vi "FindMinimumChiSquaredLMethod.vi"(0 "Extinction ExtinctionUncertainity Size parameter and Number ofS sizes 2":T2={"PAS amplitude"=[7.938e-10, 1.5399999999999999e-09, 2.52e-09, 3.6819999999999995e-09, 4.97e-09, 6.355999999999999e-09], "PAS amp Uncertainty"=[1.21e-11, 5.86e-12, 1.26e-11, 5.3e-11, 1.13e-10, 2.06e-10], "Size parameters"=[1.4957116398663945, 1.869639549832993, 2.243567459799592, 2.61749536976619, 2.991423279732789, 3.3653511896993877], "Number ofSizes"=6.0, "GeometricCrossSection"=[3.1415926535897934e-10, 4.908738521234053e-10, 7.068583470577035e-10, 9.621127501618742e-10, 1.2566370614359174e-09, 1.590431280879833e-09], "Wave Length"=420.07999, "SMPS Sizes"=[181.1, 187.7, 194.6, 200.0, 201.7, 209.1, 216.7, 224.7, 232.9, 241.4, 250.0, 250.3, 259.5, 269.0, 278.8, 289.0, 299.6, 300.0, 310.6, 322.0, 333.8, 346.0, 350.0, 358.7, 371.8, 385.4, 399.5, 400.0, 414.2, 429.4, 445.1, 450.0, 461.4, 478.3, 495.8, 514.0, 532.8, 552.3, 572.5, 593.5, 615.3, 637.8, 661.2, 685.4, 710.5, 736.5, 763.5, 791.5], "Concentration"=[[0.0, 0.0, 0.0, 1.0, 0.0, 0.0, 0.0, 0.0, 0.0, 0.0, 0.0, 0.0, 0.0, 0.0, 0.0, 0.0, 0.0, 0.0, 0.0, 0.0, 0.0, 0.0, 0.0, 0.0, 0.0, 0.0, 0.0, 0.0, 0.0, 0.0, 0.0, 0.0, 0.0, 0.0, 0.0, 0.0, 0.0, 0.0, 0.0, 0.0, 0.0, 0.0, 0.0, 0.0, 0.0, 0.0, 0.0, 0.0], [0.0, 0.0, 0.0, 0.0, 0.0, 0.0, 0.0, 0.0, 0.0, 0.0, 1.0, 0.0, 0.0, 0.0, 0.0, 0.0, 0.0, 0.0, 0.0, 0.0, 0.0, 0.0, 0.0, 0.0, 0.0, 0.0, 0.0, 0.0, 0.0, 0.0, 0.0, 0.0, 0.0, 0.0, 0.0, 0.0, 0.0, 0.0, 0.0, 0.0, 0.0, 0.0, 0.0, 0.0, 0.0, 0.0, 0.0, 0.0], [0.0, 0.0, 0.0, 0.0, 0.0, 0.0, 0.0, 0.0, 0.0, 0.0, 0.0, 0.0, 0.0, 0.0, 0.0, 0.0, 0.0, 1.0, 0.0, 0.0, 0.0, 0.0, 0.0, 0.0, 0.0, 0.0, 0.0, 0.0, 0.0, 0.0, 0.0, 0.0, 0.0, 0.0, 0.0, 0.0, 0.0, 0.0, 0.0, 0.0, 0.0, 0.0, 0.0, 0.0, 0.0, 0.0, 0.0, 0.0], [0.0, 0.0, 0.0, 0.0, 0.0, 0.0, 0.0, 0.0, 0.0, 0.0, 0.0, 0.0, 0.0, 0.0, 0.0, 0.0, 0.0, 0.0, 0.0, 0.0, 0.0, 0.0, 1.0, 0.0, 0.0, 0.0, 0.0, 0.0, 0.0, 0.0, 0.0, 0.0, 0.0, 0.0, 0.0, 0.0, 0.0, 0.0, 0.0, 0.0, 0.0, 0.0, 0.0, 0.0, 0.0, 0.0, 0.0, 0.0], [0.0, 0.0, 0.0, 0.0, 0.0, 0.0, 0.0, 0.0, 0.0, 0.0, 0.0, 0.0, 0.0, 0.0, 0.0, 0.0, 0.0, 0.0, 0.0, 0.0, 0.0, 0.0, 0.0, 0.0, 0.0, 0.0, 0.0, 1.0, 0.0, 0.0, 0.0, 0.0, 0.0, 0.0, 0.0, 0.0, 0.0, 0.0, 0.0, 0.0, 0.0, 0.0, 0.0, 0.0, 0.0, 0.0, 0.0, 0.0], [0.0, 0.0, 0.0, 0.0, 0.0, 0.0, 0.0, 0.0, 0.0, 0.0, 0.0, 0.0, 0.0, 0.0, 0.0, 0.0, 0.0, 0.0, 0.0, 0.0, 0.0, 0.0, 0.0, 0.0, 0.0, 0.0, 0.0, 0.0, 0.0, 0.0, 0.0, 1.0, 0.0, 0.0, 0.0, 0.0, 0.0, 0.0, 0.0, 0.0, 0.0, 0.0, 0.0, 0.0, 0.0, 0.0, 0.0, 0.0]], "Double Charge Correction"=TRUE, "Extincation Factor"=3.54365, "Diameter Factor"=1.0, "Diameter Offset"=0.0, "Extinction Factor Flag"=TRUE, "Diameter Factor Flag"=FALSE, "Diameter Offset Flag"=FALSE, "Sizes"=[200.0, 250.0, 300.0, 350.0, 400.0, 450.0], "ExtinctionOrAbsorptionOrScattering"=0, "Concentration(#/cc)"=[]} {"ExtinctionOrAbsorptionOrScattering" scale=0.0..2.0}, 1 "Initial Guess for Real Part":dbl=1.549732406892494 format="%#.3g", 3 "Initial Guess for Imaginary Part":dbl=0.05 format="%#.3g") -> (2 "residue":dbl=0.03850522364625282, 4 "Uncertainity in Real part":dbl=0.03896738564923848 format="%#_1g", 5 "Uncertainity in Imaginary part":dbl=0.011647008352542692 format="%#_1g", 6 "Real Part from fit":dbl=1.5413886546352171 format="%#.3g", 7 "Imaginary Part from fit":dbl=0.30769802008275493 format="%#.3g", 8 "error out":errorcluster, 9 "Extinction ExtinctionUncertainity Size parameter and Number ofS sizes 3":T2={"PAS amplitude"=[7.938e-10, 1.5399999999999999e-09, 2.52e-09, 3.6819999999999995e-09, 4.97e-09, 6.355999999999999e-09], "PAS amp Uncertainty"=[1.21e-11, 5.86e-12, 1.26e-11, 5.3e-11, 1.13e-10, 2.06e-10], "Size parameters"=[1.4957116398663945, 1.869639549832993, 2.243567459799592, 2.61749536976619, 2.991423279732789, 3.3653511896993877], "Number ofSizes"=6.0, "GeometricCrossSection"=[3.1415926535897934e-10, 4.908738521234053e-10, 7.068583470577035e-10, 9.621127501618742e-10, 1.2566370614359174e-09, 1.590431280879833e-09], "Wave Length"=420.07999, "SMPS Sizes"=[181.1, 187.7, 194.6, 200.0, 201.7, 209.1, 216.7, 224.7, 232.9, 241.4, 250.0, 250.3, 259.5, 269.0, 278.8, 289.0, 299.6, 300.0, 310.6, 322.0, 333.8, 346.0, 350.0, 358.7, 371.8, 385.4, 399.5, 400.0, 414.2, 429.4, 445.1, 450.0, 461.4, 478.3, 495.8, 514.0, 532.8, 552.3, 572.5, 593.5, 615.3, 637.8, 661.2, 685.4, 710.5, 736.5, 763.5, 791.5], "Concentration"=[[0.0, 0.0, 0.0, 1.0, 0.0, 0.0, 0.0, 0.0, 0.0, 0.0, 0.0, 0.0, 0.0, 0.0, 0.0, 0.0, 0.0, 0.0, 0.0, 0.0, 0.0, 0.0, 0.0, 0.0, 0.0, 0.0, 0.0, 0.0, 0.0, 0.0, 0.0, 0.0, 0.0, 0.0, 0.0, 0.0, 0.0, 0.0, 0.0, 0.0, 0.0, 0.0, 0.0, 0.0, 0.0, 0.0, 0.0, 0.0], [0.0, 0.0, 0.0, 0.0, 0.0, 0.0, 0.0, 0.0, 0.0, 0.0, 1.0, 0.0, 0.0, 0.0, 0.0, 0.0, 0.0, 0.0, 0.0, 0.0, 0.0, 0.0, 0.0, 0.0, 0.0, 0.0, 0.0, 0.0, 0.0, 0.0, 0.0, 0.0, 0.0, 0.0, 0.0, 0.0, 0.0, 0.0, 0.0, 0.0, 0.0, 0.0, 0.0, 0.0, 0.0, 0.0, 0.0, 0.0], [0.0, 0.0, 0.0, 0.0, 0.0, 0.0, 0.0, 0.0, 0.0, 0.0, 0.0, 0.0, 0.0, 0.0, 0.0, 0.0, 0.0, 1.0, 0.0, 0.0, 0.0, 0.0, 0.0, 0.0, 0.0, 0.0, 0.0, 0.0, 0.0, 0.0, 0.0, 0.0, 0.0, 0.0, 0.0, 0.0, 0.0, 0.0, 0.0, 0.0, 0.0, 0.0, 0.0, 0.0, 0.0, 0.0, 0.0, 0.0], [0.0, 0.0, 0.0, 0.0, 0.0, 0.0, 0.0, 0.0, 0.0, 0.0, 0.0, 0.0, 0.0, 0.0, 0.0, 0.0, 0.0, 0.0, 0.0, 0.0, 0.0, 0.0, 1.0, 0.0, 0.0, 0.0, 0.0, 0.0, 0.0, 0.0, 0.0, 0.0, 0.0, 0.0, 0.0, 0.0, 0.0, 0.0, 0.0, 0.0, 0.0, 0.0, 0.0, 0.0, 0.0, 0.0, 0.0, 0.0], [0.0, 0.0, 0.0, 0.0, 0.0, 0.0, 0.0, 0.0, 0.0, 0.0, 0.0, 0.0, 0.0, 0.0, 0.0, 0.0, 0.0, 0.0, 0.0, 0.0, 0.0, 0.0, 0.0, 0.0, 0.0, 0.0, 0.0, 1.0, 0.0, 0.0, 0.0, 0.0, 0.0, 0.0, 0.0, 0.0, 0.0, 0.0, 0.0, 0.0, 0.0, 0.0, 0.0, 0.0, 0.0, 0.0, 0.0, 0.0], [0.0, 0.0, 0.0, 0.0, 0.0, 0.0, 0.0, 0.0, 0.0, 0.0, 0.0, 0.0, 0.0, 0.0, 0.0, 0.0, 0.0, 0.0, 0.0, 0.0, 0.0, 0.0, 0.0, 0.0, 0.0, 0.0, 0.0, 0.0, 0.0, 0.0, 0.0, 1.0, 0.0, 0.0, 0.0, 0.0, 0.0, 0.0, 0.0, 0.0, 0.0, 0.0, 0.0, 0.0, 0.0, 0.0, 0.0, 0.0]], "Double Charge Correction"=TRUE, "Extincation Factor"=1.413862038778095, "Diameter Factor"=1.0, "Diameter Offset"=0.0, "Extinction Factor Flag"=TRUE, "Diameter Factor Flag"=FALSE, "Diameter Offset Flag"=FALSE, "Sizes"=[200.0, 250.0, 300.0, 350.0, 400.0, 450.0], "ExtinctionOrAbsorptionOrScattering"=0, "Concentration(#/cc)"=[]} {"ExtinctionOrAbsorptionOrScattering" scale=0.0..2.0})   [LabVIEW 2013]
uses:
  BaesDataTypeDefinition.ctl
  <vilib>/gmath/NumericalOptimization/stopping criteria.ctl
  <vilib>/gmath/NumericalOptimization/cno_bounds.ctl
  <vilib>/Analysis/6fits.llb/Curve Fitting Criteria.ctl
  <vilib>/gmath/NumericalOptimization/Downhill Simplex.vi
  <vilib>/gmath/NumericalOptimization/Nonlinear Curve Fit LM.vi
  <vilib>/gmath/NI_Gmath.lvlib
  <vilib>/Analysis/NI_AALPro.lvlib
panel:
  in  "Old":bool=TRUE
  out "number of function calls":i32=280
  out "best nonlinear fit":dbl[](array[numeric])=[7.982171035259e-10, 1.5385687168745221e-09, 2.522434483509528e-09, 3.680617366441652e-09, 4.971022260491509e-09, 6.355077797337572e-09]
  in  "stopping criteria":T1={"function tolerance"=1e-12, "parameter tolerance"=1e-06, "max iterations"=100, "max function calls"=1000, "gradient tolerance"=1e-06, "max time (sec)"=-1.0}
  out "Enum":T3(ring)=enum."ExF1DiF0DiO0"
  in  "termination":cluster{"max iteration":i32, "tolerance":dbl}={"max iteration"=1000, "tolerance"=1e-20}
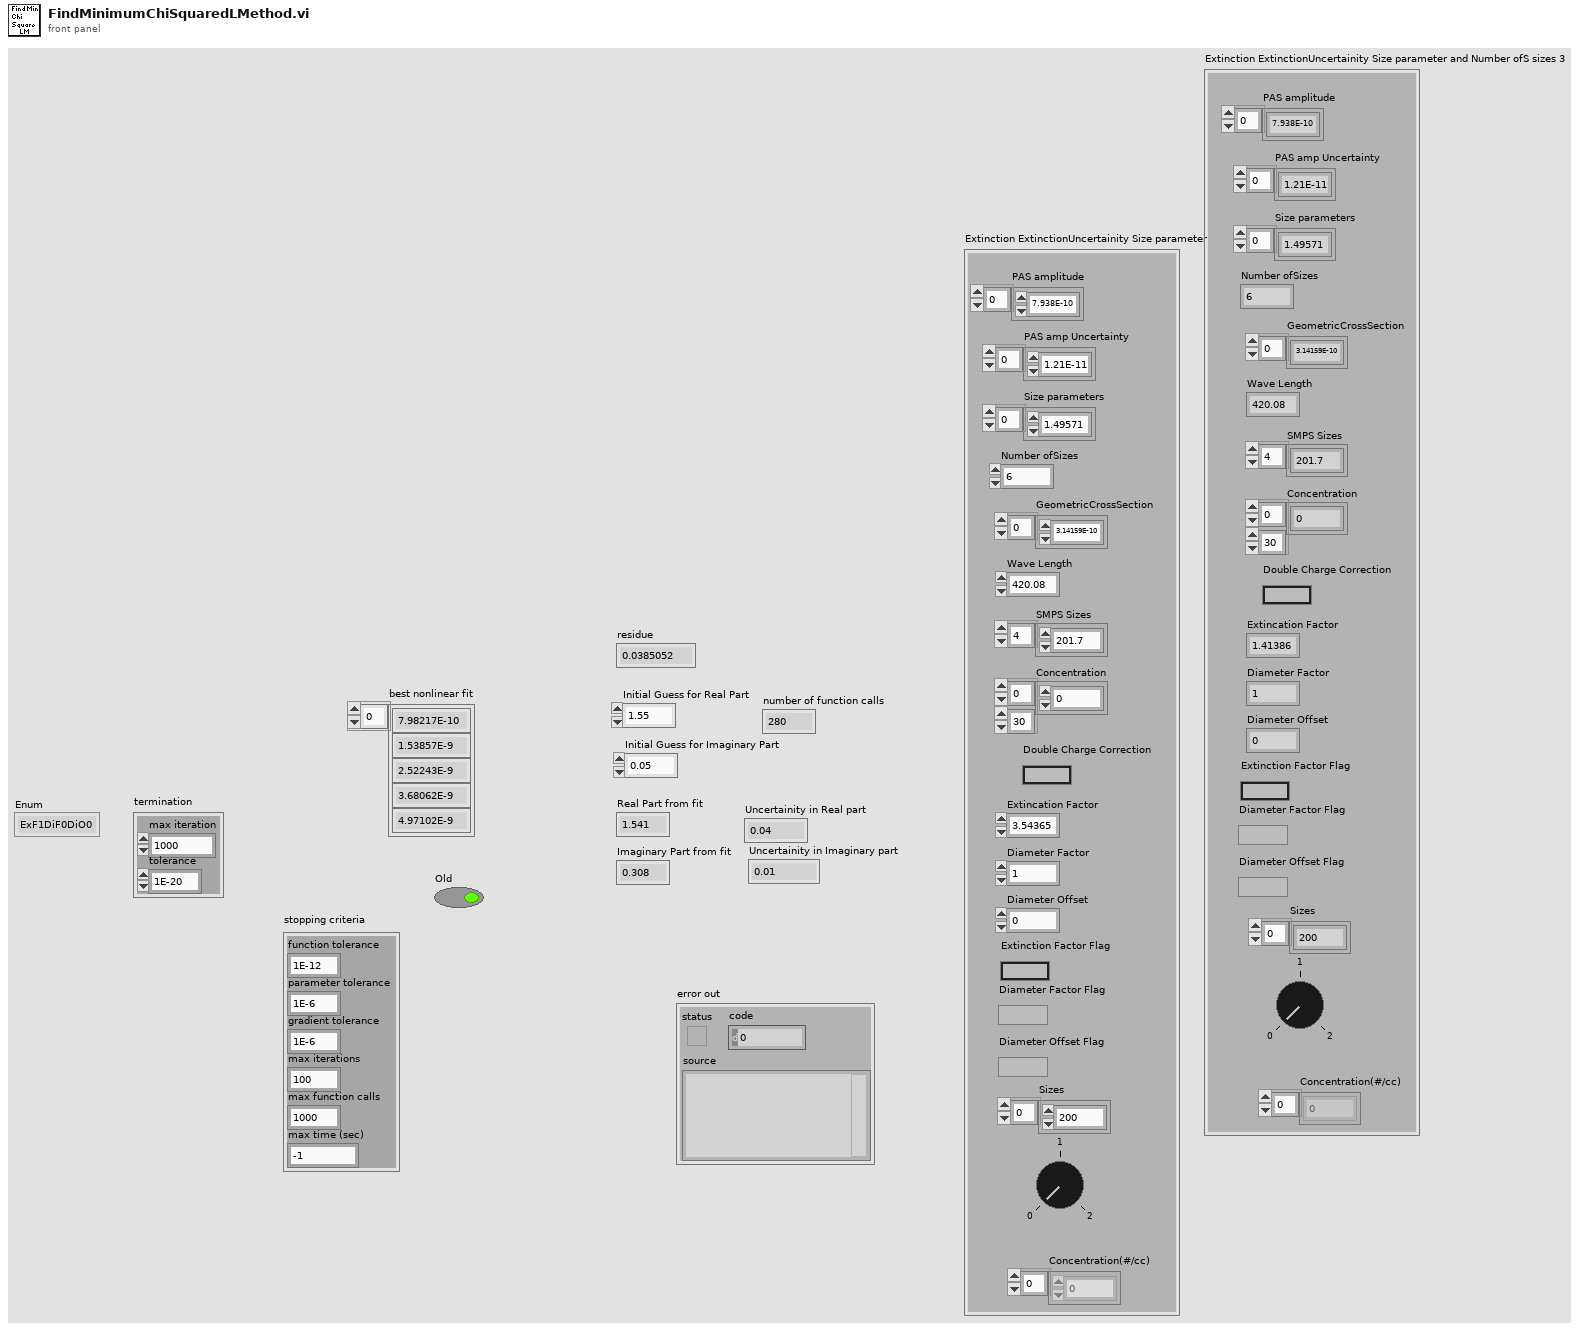
[diagram p1: front panel]
types:
  T1 = typedef "NI_Gmath.lvlib/stopping criteria.ctl" = cluster{"function tolerance":dbl, "parameter tolerance":dbl, "max iterations":i32, "max function calls":i32, "gradient tolerance":dbl, "max time (sec)":dbl}
  T2 = typedef "BaesDataTypeDefinition.ctl" = cluster{"PAS amplitude":dbl[], "PAS amp Uncertainty":dbl[], "Size parameters":dbl[], "Number ofSizes":dbl, "GeometricCrossSection":dbl[], "Wave Length":dbl, "SMPS Sizes":dbl[], "Concentration":dbl[][], "Double Charge Correction":bool, "Extincation Factor":dbl, "Diameter Factor":dbl, "Diameter Offset":dbl, "Extinction Factor Flag":bool, "Diameter Factor Flag":bool, "Diameter Offset Flag":bool, "Sizes":dbl[], "ExtinctionOrAbsorptionOrScattering":i8, "Concentration(#/cc)":dbl[]}
  T3 = enum16{"ExF0DiF0DiO0", "ExF0DiF0DiO1", "ExF0DiF1DiO0", "NotDefined1", "ExF1DiF0DiO0", "ExF1DiF0DiO1", "ExF1DiF1DiO0", "NotDefined"}
  T4 = typedef "NI_Gmath.lvlib/cno_bounds.ctl" = cluster{"X minimum":dbl[], "X maximum":dbl[], "inequality constraint minimum":dbl[], "inequality constraint maximum":dbl[]}
  T5 = typedef "NI_AALPro.lvlib/Curve Fitting Criteria.ctl" = u16
  T6 = cluster{"parameter minimum":dbl[], "parameter maximum":dbl[]}
  T7 = typedef "NI_Matrix.lvlib/RealMatrix.ctl" = dbl[][]
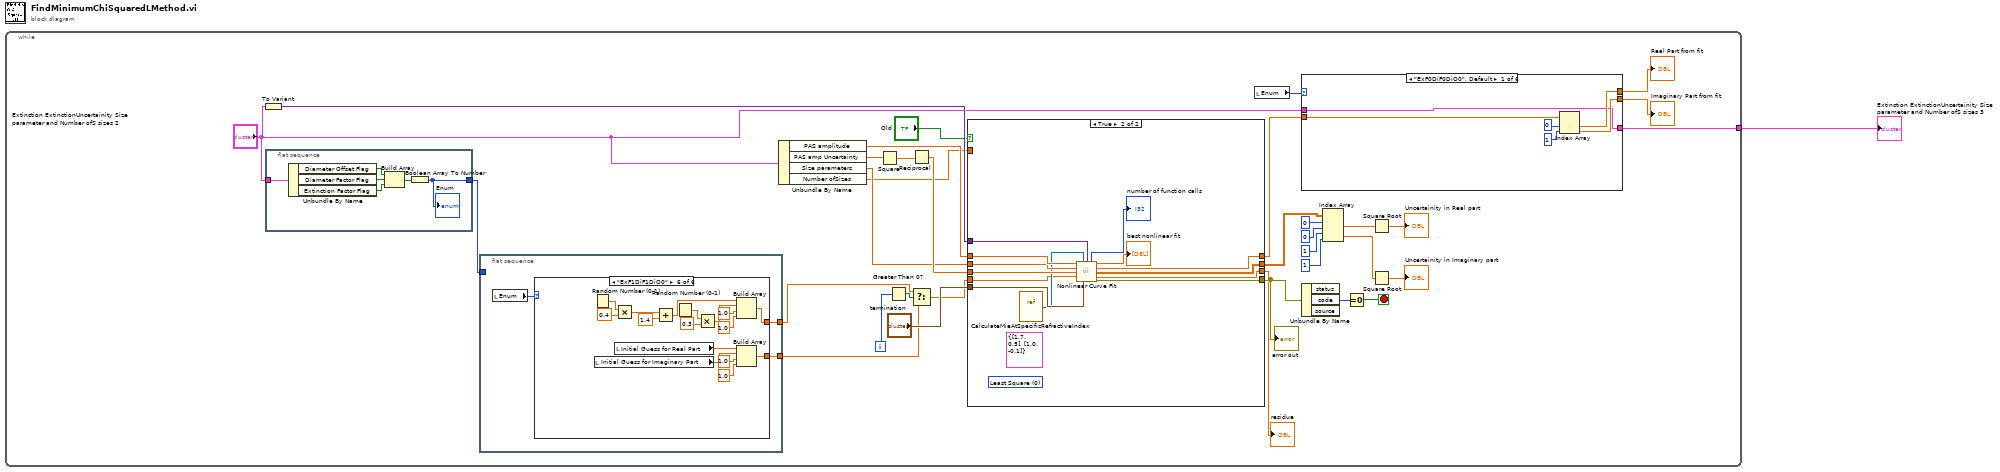
[diagram p0: block diagram]
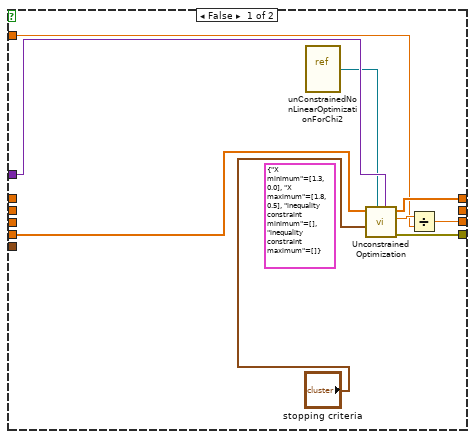
[diagram p2: hidden frame]
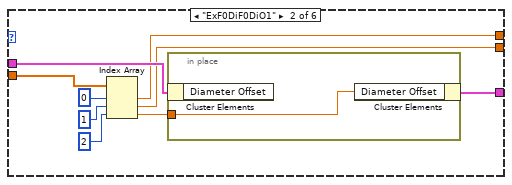
[diagram p3: hidden frame]
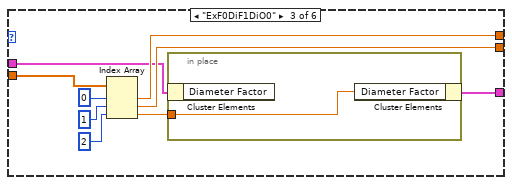
[diagram p4: hidden frame]
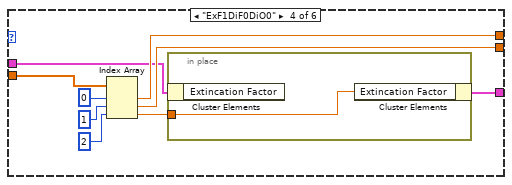
[diagram p5: hidden frame]
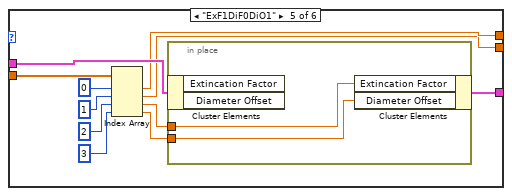
[diagram p6: hidden frame]
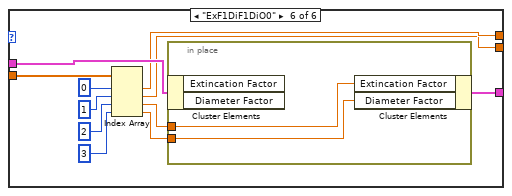
[diagram p7: hidden frame]
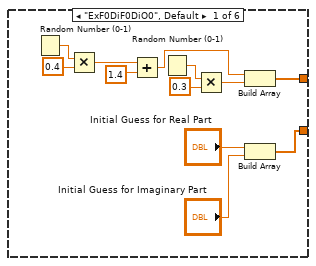
[diagram p8: hidden frame]
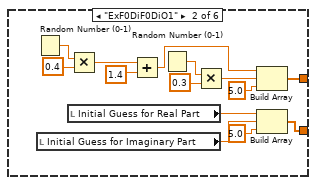
[diagram p9: hidden frame]
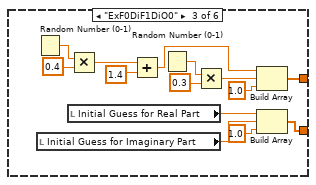
[diagram p10: hidden frame]
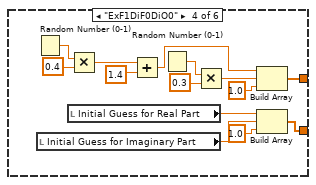
[diagram p11: hidden frame]
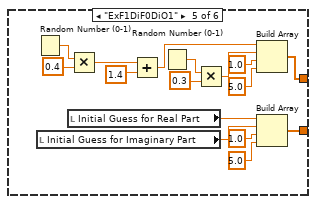
[diagram p12: hidden frame]
diagram:
  n1 = while {
    tunnel: [w5] -> w1
    i -> [w16]
    stop <- w22 stop-if-true
    n2 = To Variant(anything="Extinction ExtinctionUncertainity Size parameter and Number ofS sizes 2") -> (Variant=w18:variant)
    n3 = flat-sequence {
      tunnel: "Extinction ExtinctionUncertainity Size parameter and Number ofS sizes 2" -> [w210]
      tunnel: [w209] -> w11
      frame #0 {
        n4 = Unbundle By Name(w210) -> ("Diameter Offset Flag"=w214:bool, "Diameter Factor Flag"=w213:bool, "Extinction Factor Flag"=w212:bool)
        n5 = Build Array(w214, w213, w212) -> (w211:bool[])
        n6 = Boolean Array To Number(Boolean array=w211) -> (number=w209:u32)
        "Enum" <- w209
      }
    }
    n7 = flat-sequence {
      tunnel: [w121] -> w14
      tunnel: [w120] -> w13
      tunnel: w11 -> [_]
      frame #0 {
        n8 = local read "Enum"() -> (w122:T3)
        n9 = case shown="\"ExF1DiF1DiO0\"" w122 {
          tunnel: [w124 w135 w149 w165 w177 w193] -> w121
          tunnel: [w123 w136 w150 w166 w178 w194] -> w120
          frame "ExF0DiF0DiO0", Default {
            n10 = Random Number (0-1)() -> (number: 0 to 1=w131:dbl)
            n11 = Multiply(x=w131, y=0.4) -> (x*y=w129:dbl)
            n12 = Add(x=w129, y=1.4) -> (x+y=w127:dbl)
            n13 = Random Number (0-1)() -> (number: 0 to 1=w134:dbl)
            n14 = Multiply(x=w134, y=0.3) -> (x*y=w132:dbl)
            n15 = Build Array(w127, w132) -> (w124:dbl[])
            n16 = Build Array("Initial Guess for Real Part", "Initial Guess for Imaginary Part") -> (w123:dbl[])
          }
          frame "ExF0DiF0DiO1" {
            n17 = Random Number (0-1)() -> (number: 0 to 1=w145:dbl)
            n18 = local read "Initial Guess for Imaginary Part"() -> (w137:dbl)
            n19 = local read "Initial Guess for Real Part"() -> (w138:dbl)
            n20 = Multiply(x=w145, y=0.4) -> (x*y=w143:dbl)
            n21 = Add(x=w143, y=1.4) -> (x+y=w141:dbl)
            n22 = Random Number (0-1)() -> (number: 0 to 1=w148:dbl)
            n23 = Multiply(x=w148, y=0.3) -> (x*y=w146:dbl)
            n24 = Build Array(w141, w146, 5.0 ("element")) -> (w135:dbl[])
            n25 = Build Array(w138, w137, 5.0 ("element")) -> (w136:dbl[])
          }
          frame "ExF0DiF1DiO0" {
            n26 = Random Number (0-1)() -> (number: 0 to 1=w159:dbl)
            n27 = local read "Initial Guess for Imaginary Part"() -> (w152:dbl)
            n28 = local read "Initial Guess for Real Part"() -> (w151:dbl)
            n29 = Multiply(x=w159, y=0.4) -> (x*y=w157:dbl)
            n30 = Add(x=w157, y=1.4) -> (x+y=w155:dbl)
            n31 = Random Number (0-1)() -> (number: 0 to 1=w162:dbl)
            n32 = Multiply(x=w162, y=0.3) -> (x*y=w160:dbl)
            n33 = Build Array(w155, w160, 1.0 ("element")) -> (w149:dbl[])
            n34 = Build Array(w151, w152, 1.0 ("element")) -> (w150:dbl[])
          }
          frame "ExF1DiF0DiO0" {
            n35 = Random Number (0-1)() -> (number: 0 to 1=w173:dbl)
            n36 = local read "Initial Guess for Imaginary Part"() -> (w163:dbl)
            n37 = local read "Initial Guess for Real Part"() -> (w164:dbl)
            n38 = Multiply(x=w173, y=0.4) -> (x*y=w171:dbl)
            n39 = Add(x=w171, y=1.4) -> (x+y=w169:dbl)
            n40 = Random Number (0-1)() -> (number: 0 to 1=w176:dbl)
            n41 = Multiply(x=w176, y=0.3) -> (x*y=w174:dbl)
            n42 = Build Array(w169, w174, 1.0 ("element")) -> (w165:dbl[])
            n43 = Build Array(w164, w163, 1.0 ("element")) -> (w166:dbl[])
          }
          frame "ExF1DiF0DiO1" {
            n44 = Random Number (0-1)() -> (number: 0 to 1=w189:dbl)
            n45 = local read "Initial Guess for Imaginary Part"() -> (w181:dbl)
            n46 = local read "Initial Guess for Real Part"() -> (w182:dbl)
            n47 = Multiply(x=w189, y=0.4) -> (x*y=w187:dbl)
            n48 = Add(x=w187, y=1.4) -> (x+y=w185:dbl)
            n49 = Random Number (0-1)() -> (number: 0 to 1=w192:dbl)
            n50 = Multiply(x=w192, y=0.3) -> (x*y=w190:dbl)
            n51 = Build Array(w185, w190, 1.0 ("element"), 5.0 ("element")) -> (w177:dbl[])
            n52 = Build Array(w182, w181, 1.0 ("element"), 5.0 ("element")) -> (w178:dbl[])
          }
          frame "ExF1DiF1DiO0" {
            n53 = Random Number (0-1)() -> (number: 0 to 1=w205:dbl)
            n54 = local read "Initial Guess for Imaginary Part"() -> (w197:dbl)
            n55 = local read "Initial Guess for Real Part"() -> (w198:dbl)
            n56 = Multiply(x=w205, y=0.4) -> (x*y=w203:dbl)
            n57 = Add(x=w203, y=1.4) -> (x+y=w201:dbl)
            n58 = Random Number (0-1)() -> (number: 0 to 1=w208:dbl)
            n59 = Multiply(x=w208, y=0.3) -> (x*y=w206:dbl)
            n60 = Build Array(w201, w206, 1.0 ("element"), 1.0 ("element")) -> (w193:dbl[])
            n61 = Build Array(w198, w197, 1.0 ("element"), 1.0 ("element")) -> (w194:dbl[])
          }
        }
      }
    }
    n62 = Unbundle By Name("Extinction ExtinctionUncertainity Size parameter and Number ofS sizes 2") -> ("PAS amplitude"=w20:dbl[], "PAS amp Uncertainty"=w19:dbl[], "Size parameters"=w12:dbl[], "Number ofSizes"=w3:dbl)
    n63 = Square(x=w19) -> (x^2=w35:dbl[])
    n64 = Greater Than 0?(x=w16) -> (x > 0?=w15:bool)
    n65 = Reciprocal(x=w35) -> (1/x=w34:dbl[])
    n66 = Select(t=w14, s=w15, f=w13) -> (s? t:f=w17:dbl[])
    n67 = case shown="True" "Old" {
      tunnel: w34 -> [_ w57]
      tunnel: [_ w56] -> w33
      tunnel: [w41 w55] -> w24
      tunnel: "termination" -> [_ w54]
      tunnel: w20 -> [_ w53]
      tunnel: w18 -> [w44 w52]
      tunnel: w17 -> [w37 w47]
      tunnel: w12 -> [_ w51]
      tunnel: [w42 w50] -> w9
      tunnel: [w38 w49] -> w4
      tunnel: w3 -> [w39 _]
      frame False {
        (unwired) T4 {"X minimum"=[1.3, 0.0], "X maximum"=[1.8, 0.5], "inequality constraint minimum"=[], "inequality constraint maximum"=[]} ("bounds")
        n68 = vi-ref "unConstrainedNonLinearOptimizationForChi2.vi"() -> (w36:refnum<vi>)
        n69 = call-poly <vilib>:"Unconstrained Optimization.vi"("function data"=w44, "objective function"=w36, "stopping criteria"="stopping criteria", "start"=w37) -> ("error out"=w41:errorcluster, "f(minimum)"=w40:dbl, "minimum"=w42:dbl[])  [unwired: 4 in, 1 out]
        n70 = Divide(x=w40, y=w39) -> (x/y=w38:dbl)
      }
      frame True {
        (unwired) T5 0 items=["Least Square", "Least Absolute Residual", "Bisquare"] ("method")
        (unwired) T6 {"parameter minimum"=[1.7, 0.5], "parameter maximum"=[1.0, -0.1]} ("parameter bounds")
        n71 = vi-ref "CalculateMieAtSpecificRefractiveIndex.vi"() -> (w48:refnum<vi>)
        n72 = call-poly <vilib>:"Nonlinear Curve Fit.vi"("Y"=w53, "f(x,a)"=w48, "data"=w52, "X"=w51, "Weight"=w57, "initial parameters"=w47, "termination"=w54) -> ("number of function calls"=→"number of function calls":i32, "best nonlinear fit"=→"best nonlinear fit":dbl[], "best fit parameters"=w50:dbl[], "covariance"=w56:T7, "residue"=w49:dbl, "error out"=w55:errorcluster)  [unwired: 3 in]
      }
    }
    "error out" <- w24
    "residue" <- w4
    n73 = local read "Enum"() -> (w10:T3)
    n74 = case shown="\"ExF0DiF0DiO0\", Default" w10 {
      tunnel: w9 -> [w61 w68 w75 w89 w100 w110]
      tunnel: [w60 w65 w77 w87 w96 w108] -> w8
      tunnel: [w59 w66 w78 w88 w97 w109] -> w7
      tunnel: "Extinction ExtinctionUncertainity Size parameter and Number ofS sizes 2" -> [w58 w67 w76 w86 w99 w111]
      tunnel: [w58 w64 w74 w84 w98 w107] -> w5
      frame "ExF0DiF0DiO0", Default {
        n75 = Index Array(array=w61, index #1=0 ("index"), index #2=1 ("index")) -> (element #1=w59:dbl, element #2=w60:dbl)
      }
      frame "ExF0DiF0DiO1" {
        n76 = Index Array(array=w68, index #1=0 ("index"), index #2=1 ("index"), index #3=2 ("index")) -> (element #1=w66:dbl, element #2=w65:dbl, element #3=w69:dbl)
        n77 = in-place {
          in-place-border: w69 -> [w73]
          n78 = in-place-cluster #1(w67) -> ()  [unwired: 1 out]
          n79 = in-place-cluster #1("Diameter Offset"=w73) -> (w64:T2)
        }
      }
      frame "ExF0DiF1DiO0" {
        n80 = Index Array(array=w75, index #1=0 ("index"), index #2=1 ("index"), index #3=2 ("index")) -> (element #1=w78:dbl, element #2=w77:dbl, element #3=w79:dbl)
        n81 = in-place {
          in-place-border: w79 -> [w83]
          n82 = in-place-cluster #2(w76) -> ()  [unwired: 1 out]
          n83 = in-place-cluster #2("Diameter Factor"=w83) -> (w74:T2)
        }
      }
      frame "ExF1DiF0DiO0" {
        n84 = Index Array(array=w89, index #1=0 ("index"), index #2=1 ("index"), index #3=2 ("index")) -> (element #1=w88:dbl, element #2=w87:dbl, element #3=w85:dbl)
        n85 = in-place {
          in-place-border: w85 -> [w93]
          n86 = in-place-cluster #3(w86) -> ()  [unwired: 1 out]
          n87 = in-place-cluster #3("Extincation Factor"=w93) -> (w84:T2)
        }
      }
      frame "ExF1DiF0DiO1" {
        n88 = Index Array(array=w100, index #1=0 ("index"), index #2=1 ("index"), index #3=2 ("index"), index #4=3 ("index")) -> (element #1=w97:dbl, element #2=w96:dbl, element #3=w101:dbl, element #4=w94:dbl)
        n89 = in-place {
          in-place-border: w101 -> [w106]
          in-place-border: w94 -> [w105]
          n90 = in-place-cluster #4(w99) -> ()  [unwired: 2 out]
          n91 = in-place-cluster #4("Extincation Factor"=w106, "Diameter Offset"=w105) -> (w98:T2)
        }
      }
      frame "ExF1DiF1DiO0" {
        n92 = Index Array(array=w110, index #1=0 ("index"), index #2=1 ("index"), index #3=2 ("index"), index #4=3 ("index")) -> (element #1=w109:dbl, element #2=w108:dbl, element #3=w114:dbl, element #4=w112:dbl)
        n93 = in-place {
          in-place-border: w114 -> [w119]
          in-place-border: w112 -> [w118]
          n94 = in-place-cluster #5(w111) -> ()  [unwired: 2 out]
          n95 = in-place-cluster #5("Extincation Factor"=w119, "Diameter Factor"=w118) -> (w107:T2)
        }
      }
    }
    "Real Part from fit" <- w7
    "Imaginary Part from fit" <- w8
    n96 = Unbundle By Name(w24) -> ("code"=w23:i32)  [unwired: 2 out]
    n97 = Index Array(array=w33, index (row) #1=0 ("index (row)"), index (col) #1=0 ("index (col)"), index (row) #2=1 ("index (row)"), index (col) #2=1 ("index (col)")) -> (element #1=w28:dbl, element #2=w27:dbl)
    n98 = Equal To 0?(x=w23) -> (x = 0?=w22:bool)
    n99 = Square Root(x=w28) -> (sqrt(x)=→"Uncertainity in Real part":dbl)
    n100 = Square Root(x=w27) -> (sqrt(x)=→"Uncertainity in Imaginary part":dbl)
  }
  "Extinction ExtinctionUncertainity Size parameter and Number ofS sizes 3" <- w1
